vi "Write Fixture ID.vi"(8 "error in (no error)":errorcluster, 10 "Fixture ID":string[](array[string]), 11 "LunchTest in":refnum<class "LunchTest.lvclass">) -> (0 "error out":errorcluster, 3 "LunchTest out":refnum<class "LunchTest.lvclass">)   [LabVIEW 2019, in "SignalProcessing.lvlib" / "LunchTest.lvclass"]
uses:
  LunchTest.lvclass
  LunchTest.lvclass/LunchTest.ctl
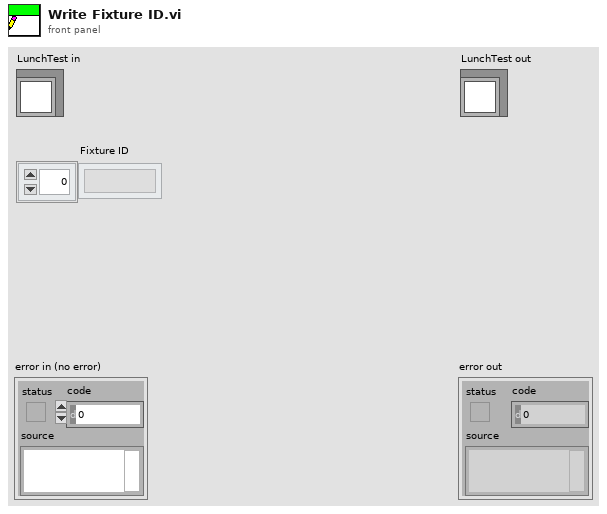
[diagram p1: front panel]
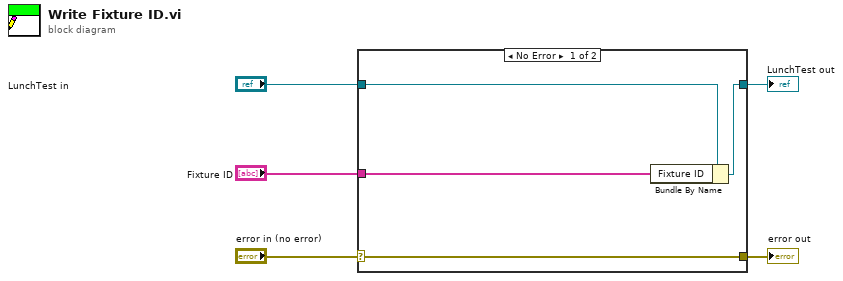
[diagram p0: block diagram]
diagram:
  n1 = case shown="No Error" "error in (no error)" {
    selector: "error in (no error)" -> [w9 w10]
    tunnel: [w9 w10] -> w4
    tunnel: [w7 w11] -> w2
    tunnel: "LunchTest in" -> [w8 w11]
    tunnel: "Fixture ID" -> [w6 _]
    frame No Error {
      n2 = Bundle By Name(cluster=w8, "Fixture ID"=w6) -> (w7:refnum<class "LunchTest.lvclass">)
    }
    frame Error {
    }
  }
  "error out" <- w4
  "LunchTest out" <- w2
